vi "Orca Flash Engine.vi"(0 "Notifier Name":string, 11 "Camera ID":string[](array[string])) -> ()   [LabVIEW 2016]
uses:
  Orca Flash Controls/Orca Flash Parameters.ctl
  Orca Flash Controls/Orca Flash Parameter List.ctl
  Orca Flash Controls/Orca Flash ROI.ctl
  Orca Flash Controls/Orca Flash Notifier Element.ctl
  Orca Flash Controls/Orca Flash Actions.ctl
  <vilib>/vision/Image Controls.llb/IMAQ Image.ctl
  Camera Controls/Camera IMAQ Key Info.ctl
panel:
  in  "Orca Flash ROI":T1
  in  "Use Display Module":bool
  in  "Sensor Mode":enum32{"Area", "Progressive"}(radio)
  in  "Number of lines":dbl=8.0
  in  "Internal Line Interval Setpoint":dbl=0.001
  in  "Get Parameter":bool
  in  "Set Parameter":bool
  in  "Get ROI":bool
  in  "Set ROI":bool
  in  "sCMOS Parameter":T2={"Value"=0.0, "Parameter"=2049184} {"Parameter" items=["SENSOR MODE"=4212128, "READOUT SPEED"=4211872, "READOUT DIRECTION"=4211904, "TRIGGER GLOBAL EXPOSURE"=2049680, "TRIGGER DELAY"=1066480, "SYNC READOUT SYSTEM BLANK"=1066528, "SENSOR COOLER"=2115248, "SENSOR COOLER STATUS"=2115280, "EXPOSURE TIME"=2049184, "DEFECT CORRECT MODE"=4670368, "BINNING"=4215968, "INTERNAL LINE SPEED"=4226000, "INTERNAL LINE INTERVAL"=4226016, "IMAGE PIXEL TYPE"=4343296, "NUMBER OF OUTPUT TRIGGER CONNECTOR"=1852320, "OUTPUT TRIGGER SOURCE[0]"=1852576, "OUTPUT TRIGGER SOURCE[1]"=1852832, "OUTPUT TRIGGER SOURCE[2]"=1853088, "OUTPUT TRIGGER POLARITY[0]"=1852592, "OUTPUT TRIGGER POLARITY[1]"=1852848, "OUTPUT TRIGGER POLARITY[2]"=1853104, "OUTPUT TRIGGER ACTIVE[0]"=1852608, "OUTPUT TRIGGER ACTIVE[1]"=1852864, "OUTPUT TRIGGER ACTIVE[2]"=1853120, "OUTPUT TRIGGER DELAY[0]"=1852624, "OUTPUT TRIGGER DELAY[1]"=1852880, "OUTPUT TRIGGER DELAY[2]"=1853136, "OUTPUT TRIGGER PERIOD[0]"=1852640, "OUTPUT TRIGGER PERIOD[1]"=1852896, "OUTPUT TRIGGER PERIOD[2]"=1853152, "OUTPUT TRIGGER KIND[0]"=1852656, "OUTPUT TRIGGER KIND[1]"=1852912, "OUTPUT TRIGGER KIND[2]"=1853168, "OUTPUT TRIGGER PRE HSYNC COUNT"=1852704]}
  in  "# of frames":i32=100
  in  "Path":path
  in  "RECORD":bool
  in  "PREVIEW":bool
  out "Acquisition Loop":i32
  in  "QUIT":bool
  out "Acquisition Frame":i32
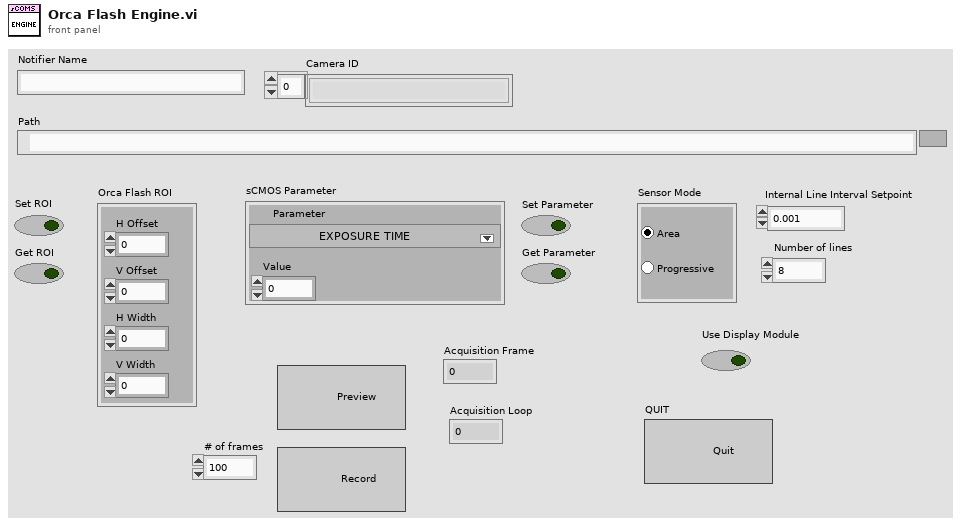
[diagram p1: front panel]
types:
  T1 = typedef "Orca Flash ROI.ctl" = cluster{"H Offset":i32, "V Offset":i32, "H Width":i32, "V Width":i32}
  T2 = typedef "Orca Flash Parameters.ctl" = cluster{"Value":dbl, "Parameter":T3}
  T3 = typedef "Orca Flash Parameter List.ctl" = u32
  T4 = typedef "Camera IMAQ Key Info.ctl" = cluster{"Frame":u32, "Sensor Height":i32, "Sensor Width":i32, "ROI Height":i32, "ROI Width":i32, "ROI Enable?":bool, "Bit per Pixel":u8}
  T5 = typedef "Image Type" = u32
  T6 = typedef "Orca Flash Notifier Element.ctl" = cluster{"Camera Actions":T7, "Received?":bool, "Running?":bool, "sCMOS Parameter":T2, "sCMOS ROI":T1, "Save Path":path, "# of frames":u32, "Image Ref":T8}
  T7 = typedef "Orca Flash Actions.ctl" = enum16{"IDLE", "PREVIEW", "RECORD", "Record Settings", "SETPARAM", "GETPARAM", "SETROI", "GETROI", "PROGRESSIVE MODE", "AREA MODE", "STATUS", "QUIT"}
  T8 = typedef "IMAQ Image.ctl" = refnum<image>
  T9 = enum32{"Invalid", "Standard", "Closed", "Hidden", "Minimized", "Maximized"}
  T10 = cluster{"Horizontal Offset":i32, "Vertical Offset":i32, "Horizontal Size":i32, "Vertical Size":i32}
  T11 = typedef "LVMinMaxIncTypeDef.ctl" = cluster{"Minimum":dbl, "Maximum":dbl, "Increment":dbl}
  T12 = cluster{"H Offset":cluster{"Value":i32, "Limits":T11}, "V Offset":cluster{"Value":i32, "Limits":T11}, "H Size":cluster{"Value":i32, "Limits":T11}, "V Size":cluster{"Value":i32, "Limits":T11}}
  T13 = cluster{"Input Trigger Mode":u32, "Input Trigger Polarity":u32, "Times":u32, "Delay":dbl}
  T14 = cluster{"Output Trigger Period":dbl, "Delay":dbl, "Source":u32}
  T15 = cluster{"Output Trigger Mode":u32, "Output Trigger Polarity":u32}
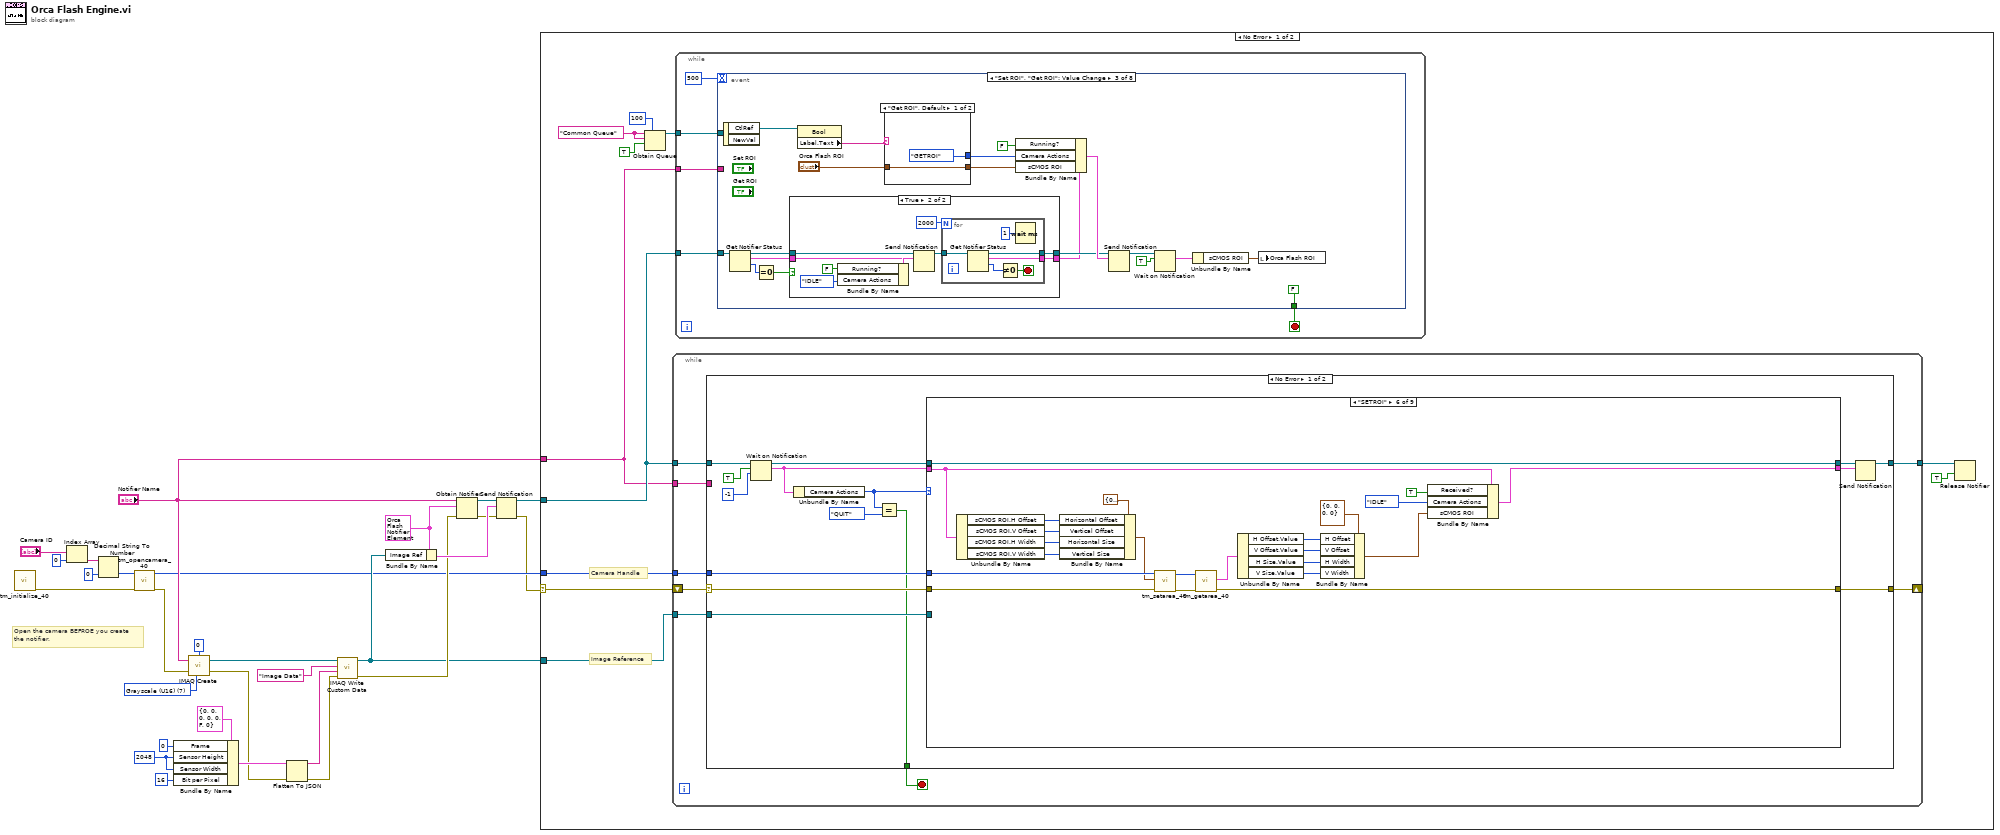
[diagram p0: block diagram]
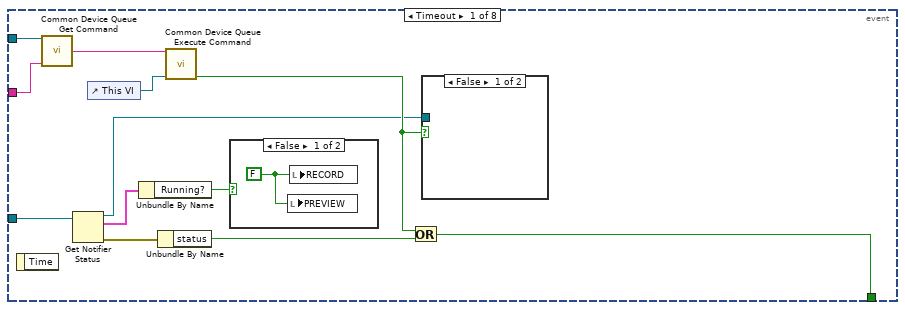
[diagram p2: hidden frame]
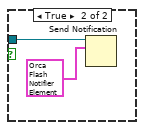
[diagram p3: hidden frame]
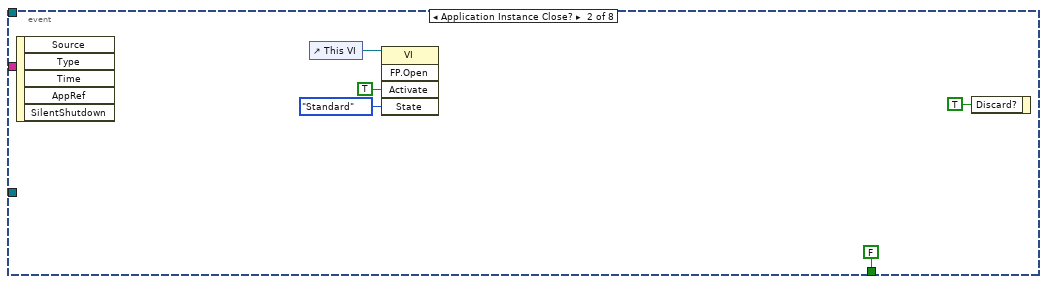
[diagram p5: hidden frame]
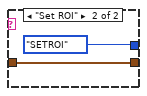
[diagram p7: hidden frame]
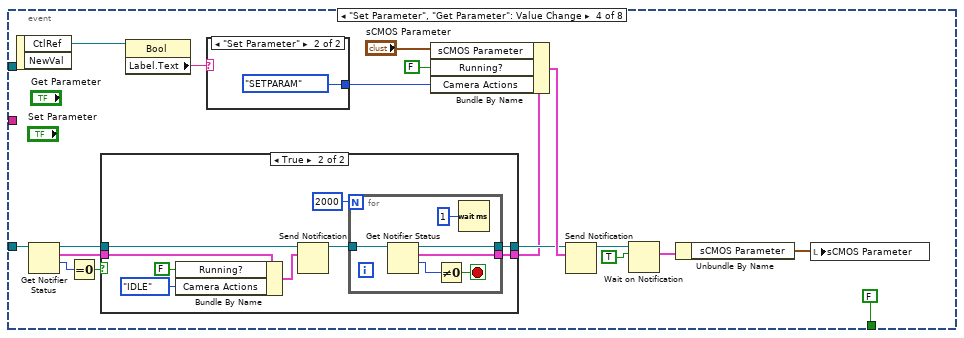
[diagram p8: hidden frame]
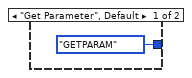
[diagram p10: hidden frame]
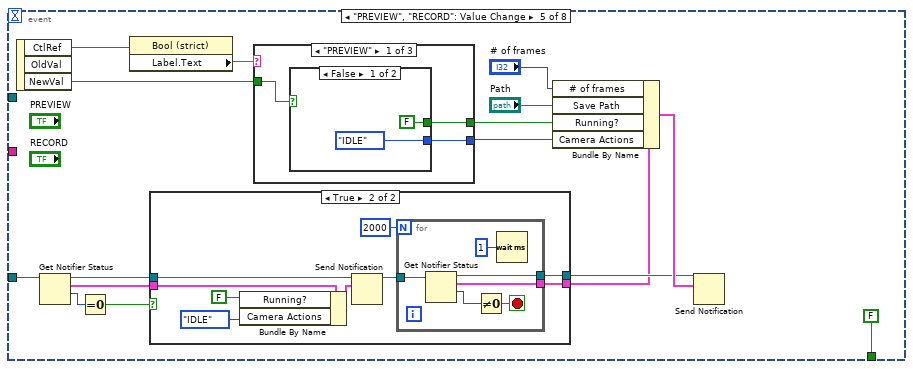
[diagram p11: hidden frame]
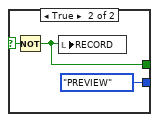
[diagram p13: hidden frame]
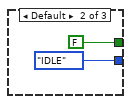
[diagram p14: hidden frame]
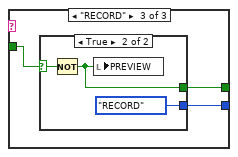
[diagram p15: hidden frame]
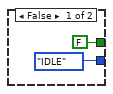
[diagram p16: hidden frame]
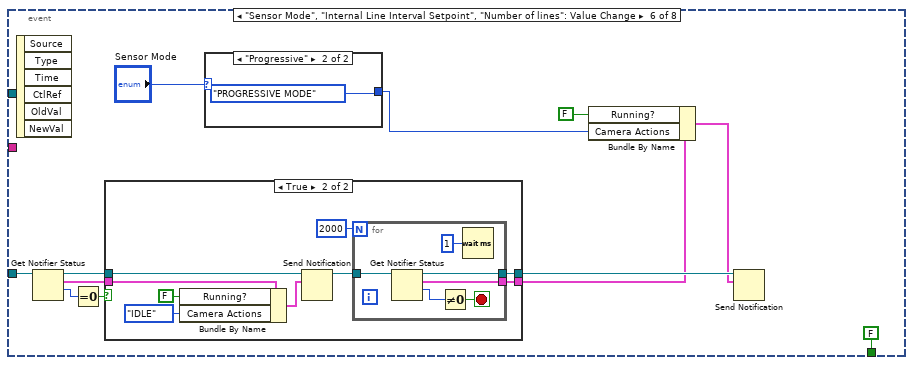
[diagram p17: hidden frame]
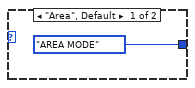
[diagram p18: hidden frame]
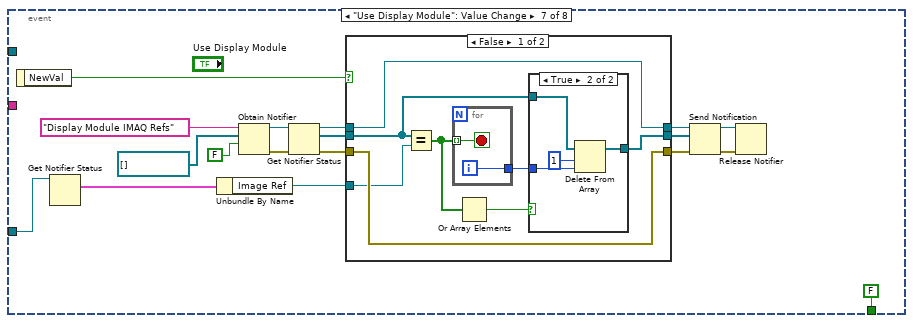
[diagram p20: hidden frame]
diagram:
  w14 = 2048 ("Sensor Height")
  w10 = T5 7 items=["Grayscale (U8)", "Grayscale (I16)", "Grayscale (SGL)", "Complex (CSG)", "RGB (U32)", "HSL (U32)", "RGB (U64)", "Grayscale (U16)"] ("Image Type")
  w24 = T6 {"Camera Actions"=enum."IDLE", "Received?"=FALSE, "Running?"=FALSE, "sCMOS Parameter"={"Value"=0.0, "Parameter"=0}, "sCMOS ROI"={"H Offset"=0, "V Offset"=0, "H Width"=0, "V Width"=0}, "Save Path"=path "", "# of frames"=1, "Image Ref"=refnum} ("Camera Cluster")
  # "Open the camera BEFROE you create\nthe notifier."
  n1 = call <userlib>:"tm_initialize_40.vi"() -> ("error out"=w21:errorcluster)  [unwired: 8 in, 3 out]
  n2 = Index Array(array="Camera ID", index=0) -> (element=w27:string)
  n3 = Decimal String To Number(string=w27, default (0L)=u32 0 ("default (0 I32)")) -> (number=w20:u32)  [unwired: 1 in, 1 out]
  n4 = call <userlib>:"tm_opencamera_40.vi"("error in (no error)"=w21, "Camera Index"=w20) -> ("error out"=w2:errorcluster, "Handle out"=w3:u32)  [unwired: 7 in, 1 out]
  n5 = Bundle By Name(cluster=T4 {"Frame"=0, "Sensor Height"=0, "Sensor Width"=0, "ROI Height"=0, "ROI Width"=0, "ROI Enable?"=FALSE, "Bit per Pixel"=0} ("Camera IMAQ Key Info"), "Frame"=u32 0, "Sensor Height"=w14, "Sensor Width"=w14, "Bit per Pixel"=u8 16) -> (w17:T4)
  n6 = call "IMAQ Create"("Border Size"=0, "Image Name"="Notifier Name", "Image Type"=w10, "error in (no error)"=w2) -> ("New Image"=w12:T8, "error out"=w9:errorcluster)  [unwired: 1 in]
  n7 = Flatten To JSON(anything=w17, error in (no error)=w9) -> (JSON string=w18:string, 11:w8:errorcluster)  [unwired: 1 in]
  n8 = call "IMAQ Write Custom Data"("error in (no error)"=w8, "Custom Data In"=w18, "Key"="Image Data", "Image"=w12) -> ("error out"=w7:errorcluster, "Image Out"=w4:T8)  [unwired: 6 in]
  n9 = Bundle By Name(cluster=w24, "Image Ref"=w4) -> (w25:T6)
  n10 = Obtain Notifier(name (unnamed)="Notifier Name", notification data type=w24, error in (no error)=w7) -> (notifier out=w23:refnum<notifier>, error out=w22:errorcluster)  [unwired: 1 in, 1 out]
  n11 = Send Notification(notification=w25, notifier=w23, error in (no error)=w22) -> (notifier out=w6:refnum<notifier>, error out=w1:errorcluster)
  n12 = case shown="No Error" w1 {
    selector: w1 -> [w35 w591]
    tunnel: w6 -> [w33 w584]
    tunnel: "Notifier Name" -> [w30 w581]
    tunnel: w4 -> [w36 _]
    tunnel: w3 -> [w34 _]
    frame No Error {
      w40 = "Common Queue" ("Unique Notifier Name")
      # "Image Reference"
      # "Camera Handle"
      n13 = Obtain Queue(max queue size (-1, unlimited)=100, name (unnamed)=w40, element data type=w40, create if not found? (T)=TRUE) -> (queue out=w37:refnum<queue>)  [unwired: 1 in, 2 out]
      n14 = while {
        tunnel: w33 -> [w298]
        tunnel: w36 -> [w297]
        shift-right: [w295] -> _
        shift-left: w35 -> [w294]
        tunnel: w34 -> [w296]
        tunnel: [w293] -> w31
        tunnel: w30 -> [w291]
        stop <- w292 stop-if-true
        n15 = case shown="No Error" w294 {
          selector: w294 -> [w303 w572]
          tunnel: w298 -> [w313 w580]
          tunnel: w297 -> [w312 _]
          tunnel: [w302 w580] -> w293
          tunnel: w296 -> [w305 _]
          tunnel: [w304 errorcluster {"status"=FALSE, "code"=0, "source"=""} ("error out")] -> w295
          tunnel: [w299 FALSE] -> w292
          tunnel: w291 -> [_ w571]
          frame No Error {
            n16 = Wait on Notification(notifier=w313, ignore previous (F)=TRUE, timeout in ms (-1)=-1) -> (notifier out=w308:refnum<notifier>, notification=w307:T6)  [unwired: 1 in, 2 out]
            n17 = Unbundle By Name(w307) -> ("Camera Actions"=w301:T7)
            n18 = Equal?(x=w301, y=Orca_Flash_Actions."QUIT") -> (x = y?=w299:bool)
            n19 = case shown="\"SETROI\"" w301 {
              selector: w301 -> [_ w321 _ _ _ _ _ _ _]
              tunnel: w305 -> [_ w346 w423 w439 w452 w475 w486 w507 w561]
              tunnel: w303 -> [w318 w325 w424 w438 w451 w474 w485 w506 w560]
              tunnel: [w318 w330 w422 w434 w450 w467 w484 w494 w550] -> w304
              tunnel: w308 -> [w317 w353 w430 w443 w453 w476 w491 w521 w570]
              tunnel: w312 -> [_ w344 w425 _ _ _ _ _ _]
              tunnel: w307 -> [w315 w342 w428 w437 w448 w470 w488 w518 w557]
              tunnel: [w317 w343 w430 w443 w453 w476 w491 w521 w570] -> w309
              tunnel: [w314 w338 w427 w442 w444 w469 w487 w517 w556] -> w306
              frame "IDLE", Default {
                w316 = FALSE ("Running?")
                n20 = Bundle By Name(cluster=w315, "Received?"=w316, "Running?"=w316) -> (w314:T6)
              }
              frame "PREVIEW", "RECORD" {
                w319 = TRUE ("Running?")
                w350 = 1 items=["Snap", "Sequence"] ("Capture mode")
                n21 = Unbundle By Name(w342) -> ("# of frames"=w331:u32, "Save Path"=w328:path)
                n22 = Equal?(x=w321, y=Orca_Flash_Actions."RECORD") -> (x = y?=w320:bool)
                n23 = To Long Integer(number=w331) -> (32bit integer=w326:i32)
                n24 = call <userlib>:"tm_preparecapture_40.vi"("error in (no error)"=w325, "Capture mode"=w350, "Handle in"=w346) -> ("error out"=w352:errorcluster, "Handle out"=w351:u32)  [unwired: 5 in, 2 out]
                n25 = call "Orca Flash Sort Filenames.vi"("Requested File Path"=w328) -> ("Resulting File Path"=w327:path)  [unwired: 14 in]
                n26 = case shown="True" w320 {
                  tunnel: w352 -> [w355 w361]
                  tunnel: w351 -> [w354 w360]
                  tunnel: [w354 w359] -> w337
                  tunnel: [w355 w358] -> w335
                  tunnel: w327 -> [_ w357]
                  tunnel: w326 -> [_ w356]
                  frame False {
                  }
                  frame True {
                    n27 = call <userlib>:"tm_startrecorder_40.vi"("error in (no error)"=w361, "frames"=w356, "File"=w357, "Handle in"=w360) -> ("error out"=w358:errorcluster, "Handle out"=w359:u32)  [unwired: 6 in]
                  }
                }
                n28 = Bundle By Name(cluster=w342, "Running?"=w319, "Received?"=w319) -> (w341:T6)
                n29 = call <userlib>:"tm_startcapture_40.vi"("error in (no error)"=w335, "Handle in"=w337) -> ("error out"=w324:errorcluster, "Handle out"=w336:u32)  [unwired: 8 in]
                n30 = Send Notification(notification=w341, notifier=w353, error in (no error)=w324) -> (notifier out=w345:refnum<notifier>, error out=w323:errorcluster)
                n31 = case shown="No Error" w323 {
                  selector: w323 -> [w369 w419]
                  tunnel: [w377 w420] -> w349
                  tunnel: w345 -> [w376 w421]
                  tunnel: w344 -> [w375 _]
                  tunnel: [w374 w418] -> w343
                  tunnel: [w373 w417] -> w340
                  tunnel: w336 -> [w372 w420]
                  tunnel: [w371 w419] -> w334
                  tunnel: w326 -> [w370 _]
                  tunnel: w320 -> [w368 _]
                  frame No Error {
                    n32 = while {
                      tunnel: w370 -> [w405]
                      tunnel: w376 -> [w408]
                      tunnel: [w407] -> w374
                      tunnel: w375 -> [w404]
                      tunnel: [w402] -> w373
                      tunnel: w369 -> [w411]
                      tunnel: [w379] -> w371
                      tunnel: w372 -> [w412]
                      tunnel: [w400] -> w377
                      tunnel: w368 -> [w378]
                      i -> [w406]
                      stop <- w409 stop-if-true
                      w385 = "Image Data" ("Key")
                      n33 = call <userlib>:"tm_waitnextframe_40.vi"("error in (no error)"=w411, "Handle in"=w412) -> ("error out"=w396:errorcluster, "Frame Count"=w394:i32, "Frame Index"=w399:i32, "Handle out"=w410:u32)  [unwired: 6 in]
                      "Acquisition Frame" <- w394
                      n34 = call <userlib>:"tm_getframe16_40.vi"("error in (no error)"=w396, "Frame Index"=w399, "Handle in"=w410) -> ("error out"=w384:errorcluster, "Data"=w395:u16[][], "Handle out"=w400:u32)  [unwired: 5 in, 1 out]
                      n35 = case shown="False" w378 {
                        selector: w378 -> [w413 _]
                        tunnel: w405 -> [_ w416]
                        tunnel: [w413 w415] -> w397
                        tunnel: w394 -> [_ w414]
                        frame False {
                        }
                        frame True {
                          n36 = Greater Or Equal?(x=w414, y=w416) -> (x >= y?=w415:bool)
                        }
                      }
                      n37 = To Unsigned Long Integer(number=w394) -> (unsigned 32bit integer=w388:u32)
                      n38 = call "IMAQ ArrayToImage"("Image Pixels (U16)"=w395, "error in (no error)"=w384, "Image"=w404) -> ("error out"=w383:errorcluster, "Image Out"=w393:T8)  [unwired: 7 in]
                      n39 = call "IMAQ Read Custom Data"("error in (no error)"=w383, "Key"=w385, "Image"=w393) -> ("error out"=w382:errorcluster, "Custom Data Out"=w390:string, "Image (duplicate)"=w392:T8)  [unwired: 6 in]
                      n40 = Unflatten From JSON(JSON string=w390, type and defaults=T4 {"Frame"=0, "Sensor Height"=0, "Sensor Width"=0, "ROI Height"=0, "ROI Width"=0, "ROI Enable?"=FALSE, "Bit per Pixel"=0} ("Camera IMAQ Key Info"), error in (no error)=w382) -> (value=w389:T4, error out=w381:errorcluster)  [unwired: 4 in]
                      n41 = Bundle By Name(cluster=w389, "Frame"=w388) -> (w387:T4)
                      n42 = Get Notifier Status(notifier=w408) -> (notifier out=w407:refnum<notifier>, current notification=w402:T6)  [unwired: 1 in, 3 out]
                      n43 = Flatten To JSON(anything=w387, error in (no error)=w381) -> (JSON string=w386:string, 11:w380:errorcluster)  [unwired: 1 in]
                      n44 = Unbundle By Name(w402) -> ("Running?"=w403:bool)
                      n45 = call "IMAQ Write Custom Data"("error in (no error)"=w380, "Custom Data In"=w386, "Key"=w385, "Image"=w392) -> ("error out"=w379:errorcluster)  [unwired: 6 in, 1 out]
                      n46 = Unbundle By Name(w379) -> ("status"=w398:bool)
                      n47 = Not(x=w403) -> (.not. x?=w401:bool)
                      n48 = Compound Arithmetic op=OR(w401, w397, w398) -> (w409:bool)
                      "Acquisition Loop" <- w406
                    }
                  }
                  frame Error {
                    n49 = Get Notifier Status(notifier=w421) -> (notifier out=w418:refnum<notifier>, current notification=w417:T6)  [unwired: 1 in, 3 out]
                  }
                }
                n50 = call <userlib>:"tm_stopcapture_40.vi"("error in (no error)"=w334, "Handle in"=w349) -> ("error out"=w333:errorcluster, "Handle out"=w348:u32)  [unwired: 8 in]
                n51 = case shown="False" w320 {
                  tunnel: w348 -> [w363 w367]
                  tunnel: [w363 w366] -> w347
                  tunnel: w333 -> [w362 w365]
                  tunnel: [w362 w364] -> w332
                  frame False {
                  }
                  frame True {
                    n52 = call <userlib>:"tm_stoprecorder_40.vi"("error in (no error)"=w365, "Handle in"=w367) -> ("error out"=w364:errorcluster, "Handle out"=w366:u32)  [unwired: 8 in]
                  }
                }
                n53 = Bundle By Name(cluster=w340, "Running?"=FALSE, "Camera Actions"=Orca_Flash_Actions."IDLE") -> (w338:T6)
                n54 = call <userlib>:"tm_unpreparecapture_40.vi"("error in (no error)"=w332, "Handle in"=w347) -> ("error out"=w330:errorcluster)  [unwired: 8 in, 1 out]
              }
              frame "QUIT" {
                n55 = call <userlib>:"tm_closecamera_40.vi"("error in (no error)"=w424, "Handle in"=w423) -> ("error out"=w426:errorcluster)  [unwired: 9 in]
                n56 = call "IMAQ Dispose"("Image"=w425) -> ()  [unwired: 5 in, 1 out]
                n57 = Bundle By Name(cluster=w428, "Received?"=TRUE ("Running?")) -> (w427:T6)
                n58 = call <userlib>:"tm_deinitialize_40.vi"("error in (no error)"=w426) -> ("error out"=w422:errorcluster)  [unwired: 10 in]
              }
              frame "SETPARAM" {
                n59 = Unbundle By Name(w437) -> ("sCMOS Parameter.Parameter"=w432:T3, "sCMOS Parameter.Value"=w436:dbl)
                n60 = call <userlib>:"tm_setparameter_40.vi"("error in (no error)"=w438, "Value in"=w436, "Parameter"=w432, "Handle in"=w439) -> ("error out"=w435:errorcluster, "Handle out"=w433:u32)  [unwired: 6 in]
                n61 = call <userlib>:"tm_getparameter_40.vi"("error in (no error)"=w435, "Parameter"=w432, "Handle in"=w433) -> ("error out"=w434:errorcluster, "Value out"=w431:dbl)  [unwired: 6 in, 1 out]
                n62 = Bundle By Name(cluster=w437, "Received?"=TRUE ("Running?"), "Camera Actions"=Orca_Flash_Actions."IDLE", "sCMOS Parameter.Value"=w431) -> (w442:T6)
              }
              frame "GETPARAM" {
                n63 = Unbundle By Name(w448) -> ("sCMOS Parameter.Parameter"=w449:T3)
                n64 = call <userlib>:"tm_getparameter_40.vi"("error in (no error)"=w451, "Parameter"=w449, "Handle in"=w452) -> ("error out"=w450:errorcluster, "Value out"=w445:dbl)  [unwired: 6 in, 1 out]
                n65 = Bundle By Name(cluster=w448, "Received?"=TRUE ("Running?"), "Camera Actions"=Orca_Flash_Actions."IDLE", "sCMOS Parameter.Value"=w445) -> (w444:T6)
              }
              frame "SETROI" {
                n66 = Unbundle By Name(w470) -> ("sCMOS ROI.H Offset"=w455:i32, "sCMOS ROI.V Offset"=w456:i32, "sCMOS ROI.H Width"=w457:i32, "sCMOS ROI.V Width"=w458:i32)
                n67 = Bundle By Name(cluster=T10 {"Horizontal Offset"=0, "Vertical Offset"=0, "Horizontal Size"=0, "Vertical Size"=0} ("Sub Region"), "Horizontal Offset"=w455, "Vertical Offset"=w456, "Horizontal Size"=w457, "Vertical Size"=w458) -> (w454:T10)
                n68 = call <userlib>:"tm_setarea_40.vi"("error in (no error)"=w474, "Sub Region"=w454, "Handle in"=w475) -> ("error out"=w468:errorcluster, "Handle out"=w473:u32)  [unwired: 7 in]
                n69 = call <userlib>:"tm_getarea_40.vi"("error in (no error)"=w468, "Handle in"=w473) -> ("error out"=w467:errorcluster, "Sub Region"=w466:T12)  [unwired: 7 in, 1 out]
                n70 = Unbundle By Name(w466) -> ("H Offset.Value"=w464:i32, "V Offset.Value"=w463:i32, "H Size.Value"=w462:i32, "V Size.Value"=w461:i32)
                n71 = Bundle By Name(cluster=T1 {"H Offset"=0, "V Offset"=0, "H Width"=0, "V Width"=0} ("Orca Flash ROI"), "H Offset"=w464, "V Offset"=w463, "H Width"=w462, "V Width"=w461) -> (w460:T1)
                n72 = Bundle By Name(cluster=w470, "Received?"=TRUE ("Running?"), "Camera Actions"=Orca_Flash_Actions."IDLE", "sCMOS ROI"=w460) -> (w469:T6)
              }
              frame "GETROI" {
                n73 = call <userlib>:"tm_getarea_40.vi"("error in (no error)"=w485, "Handle in"=w486) -> ("error out"=w484:errorcluster, "Sub Region"=w483:T12)  [unwired: 7 in, 1 out]
                n74 = Unbundle By Name(w483) -> ("H Offset.Value"=w478:i32, "V Offset.Value"=w479:i32, "H Size.Value"=w480:i32, "V Size.Value"=w481:i32)
                n75 = Bundle By Name(cluster=T1 {"H Offset"=0, "V Offset"=0, "H Width"=0, "V Width"=0} ("Orca Flash ROI"), "H Offset"=w478, "V Offset"=w479, "H Width"=w480, "V Width"=w481) -> (w477:T1)
                n76 = Bundle By Name(cluster=w488, "Received?"=TRUE ("Running?"), "Camera Actions"=Orca_Flash_Actions."IDLE", "sCMOS ROI"=w477) -> (w487:T6)
              }
              frame "PROGRESSIVE MODE" {
                w493 = u32 2049184 items=["SENSOR MODE"=4212128, "READOUT SPEED"=4211872, "READOUT DIRECTION"=4211904, "TRIGGER GLOBAL EXPOSURE"=2049680, "TRIGGER DELAY"=1066480, "INTERNAL TRIGGER HANDLING"=1066496, "SYNC READOUT SYSTEM BLANK"=1066528, "SENSOR TEMPERATURE"=2115232, "SENSOR COOLER STATUS"=2115280, "EXPOSURE TIME"=2049184, "DEFECT CORRECT MODE"=4670368, "BINNING"=4215968, "INTERNAL LINE SPEED"=4226000, "INTERNAL LINE INTERVAL"=4226016, "NUMBER OF OUTPUT TRIGGER CONNECTOR"=1852320, "OUTPUT TRIGGER SOURCE[0]"=1852576, "OUTPUT TRIGGER SOURCE[1]"=1852832, "OUTPUT TRIGGER SOURCE[2]"=1853088, "OUTPUT TRIGGER POLARITY[0]"=1852592, "OUTPUT TRIGGER POLARITY[1]"=1852848, "OUTPUT TRIGGER POLARITY[2]"=1853104, "OUTPUT TRIGGER ACTIVE[0]"=1852608, "OUTPUT TRIGGER ACTIVE[1]"=1852864, "OUTPUT TRIGGER ACTIVE[2]"=1853120, "OUTPUT TRIGGER DELAY[0]"=1852624, "OUTPUT TRIGGER DELAY[1]"=1852880, "OUTPUT TRIGGER DELAY[2]"=1853136, "OUTPUT TRIGGER PERIOD[0]"=1852640, "OUTPUT TRIGGER PERIOD[1]"=1852896, "OUTPUT TRIGGER PERIOD[2]"=1853152, "OUTPUT TRIGGER KIND[0]"=1852656, "OUTPUT TRIGGER KIND[1]"=1852912, "OUTPUT TRIGGER KIND[2]"=1853168, "OUTPUT TRIGGER BASE SENSOR[0]"=1852672, "OUTPUT TRIGGER BASE SENSOR[1]"=1852928, "OUTPUT TRIGGER BASE SENSOR[2]"=1853184, "OUTPUT TRIGGER PRE HSYNC COUNT"=1852704] ("Parameter")
                w499 = u32 4226016 items=["SENSOR MODE"=4212128, "READOUT SPEED"=4211872, "READOUT DIRECTION"=4211904, "TRIGGER GLOBAL EXPOSURE"=2049680, "TRIGGER DELAY"=1066480, "INTERNAL TRIGGER HANDLING"=1066496, "SYNC READOUT SYSTEM BLANK"=1066528, "SENSOR TEMPERATURE"=2115232, "SENSOR COOLER STATUS"=2115280, "EXPOSURE TIME"=2049184, "DEFECT CORRECT MODE"=4670368, "BINNING"=4215968, "INTERNAL LINE SPEED"=4226000, "INTERNAL LINE INTERVAL"=4226016, "NUMBER OF OUTPUT TRIGGER CONNECTOR"=1852320, "OUTPUT TRIGGER SOURCE[0]"=1852576, "OUTPUT TRIGGER SOURCE[1]"=1852832, "OUTPUT TRIGGER SOURCE[2]"=1853088, "OUTPUT TRIGGER POLARITY[0]"=1852592, "OUTPUT TRIGGER POLARITY[1]"=1852848, "OUTPUT TRIGGER POLARITY[2]"=1853104, "OUTPUT TRIGGER ACTIVE[0]"=1852608, "OUTPUT TRIGGER ACTIVE[1]"=1852864, "OUTPUT TRIGGER ACTIVE[2]"=1853120, "OUTPUT TRIGGER DELAY[0]"=1852624, "OUTPUT TRIGGER DELAY[1]"=1852880, "OUTPUT TRIGGER DELAY[2]"=1853136, "OUTPUT TRIGGER PERIOD[0]"=1852640, "OUTPUT TRIGGER PERIOD[1]"=1852896, "OUTPUT TRIGGER PERIOD[2]"=1853152, "OUTPUT TRIGGER KIND[0]"=1852656, "OUTPUT TRIGGER KIND[1]"=1852912, "OUTPUT TRIGGER KIND[2]"=1853168, "OUTPUT TRIGGER BASE SENSOR[0]"=1852672, "OUTPUT TRIGGER BASE SENSOR[1]"=1852928, "OUTPUT TRIGGER BASE SENSOR[2]"=1853184, "OUTPUT TRIGGER PRE HSYNC COUNT"=1852704] ("Parameter")
                w510 = u32 1 items=["FORWARD"=1, "BACKWARD"=2] ("Readout Direction")
                w514 = u32 4212128 items=["SENSOR MODE"=4212128, "CCD MODE"=4212384, "READOUT MODE"=4211872, "ACTIVE VIEW INDEX"=4343136, "BITS PER CHANNEL"=4342976, "IMAGE PIXEL TYPE"=4343296, "BINNING"=4215968, "EXPOSURE TIME"=2049184, "CONTRAST GAIN"=3163312, "CONTRAST OFFSET"=3163328, "LIGHT MODE"=2114720, "SENSITIVITY"=2114992, "PHOTON IMAGING MODE"=2115200, "HIGH DYNAMIC RANGE MODE"=3163360, "WHITE BALANCE"=3163568, "TEMPERATURE"=2115232, "TEMPERATURE TARGET"=2115264, "SENSOR COOLER FAN"=2115296, "LINEBUNDLE HEIGHT"=4212192, "MECHANICAL SHUTTER"=2115488, "BACK FOCUS POSITION"=8422304, "TRIGGER CONNECTOR"=1066432, "TRIGGER SOURCE"=1066144, "OUTPUT TRIGGER SOURCE"=1852576, "TRIGGER GLOBAL EXPOSURE"=2049680, "FIRST TRIGGER BEHAVIOR"=2049696, "CHANNEL SYNC"=1852352, "READOUT DIRECTION"=4211904, "PRE HSYNC COUNT"=1852704, "INTERNAL LINE SPEED"=4191408, "INTERNAL LINE INTERVAL"=4191424] ("Parameter")
                w513 = u32 4211904 items=["SENSOR MODE"=4212128, "CCD MODE"=4212384, "READOUT MODE"=4211872, "ACTIVE VIEW INDEX"=4343136, "BITS PER CHANNEL"=4342976, "IMAGE PIXEL TYPE"=4343296, "BINNING"=4215968, "EXPOSURE TIME"=2049184, "CONTRAST GAIN"=3163312, "CONTRAST OFFSET"=3163328, "LIGHT MODE"=2114720, "SENSITIVITY"=2114992, "PHOTON IMAGING MODE"=2115200, "HIGH DYNAMIC RANGE MODE"=3163360, "WHITE BALANCE"=3163568, "TEMPERATURE"=2115232, "TEMPERATURE TARGET"=2115264, "SENSOR COOLER FAN"=2115296, "LINEBUNDLE HEIGHT"=4212192, "MECHANICAL SHUTTER"=2115488, "BACK FOCUS POSITION"=8422304, "TRIGGER CONNECTOR"=1066432, "TRIGGER SOURCE"=1066144, "OUTPUT TRIGGER SOURCE"=1852576, "TRIGGER GLOBAL EXPOSURE"=2049680, "FIRST TRIGGER BEHAVIOR"=2049696, "CHANNEL SYNC"=1852352, "READOUT DIRECTION"=4211904, "PRE HSYNC COUNT"=1852704, "INTERNAL LINE SPEED"=4191408, "INTERNAL LINE INTERVAL"=4191424] ("Parameter")
                n77 = case shown="\"Master\"" enum16{"Master", "Slave"}."Master" ("Camera Trigger Mode") {
                  tunnel: [w525 w541] -> w512
                  tunnel: [w524 w539] -> w511
                  tunnel: w507 -> [w523 w543]
                  tunnel: w506 -> [w522 w542]
                  frame "Slave", Default {
                    w530 = u32 2 items=["NEGATIVE"=1, "POSITIVE"=2] ("Input Trigger Polarity")
                    w529 = u32 2 items=["INTERNAL"=1, "EXTERNAL EDGE"=2, "EXTERNAL LEVEL"=4, "SOFTWARE"=32, "FAST REPETITION"=64, "TDI"=128, "START"=512, "SYNC READOUT"=1024] ("Input Trigger Mode")
                    n78 = Bundle("Input Trigger Mode"=w529, "Input Trigger Polarity"=w530, "Times"=u32 1, "Delay"=0.0) -> (w526:T13)  [unwired: 1 in]
                    n79 = call <userlib>:"tm_setinputtrigger_40.vi"("error in (no error)"=w522, "Parameters"=w526, "Handle in"=w523) -> ("error out"=w524:errorcluster, "Handle out"=w525:u32)  [unwired: 7 in]
                  }
                  frame "Master" {
                    w536 = u32 2 items=["Exposure"=1, "Readout End"=2, "V Sync"=3, "H Sync"=4, "Trigger"=6] ("Source")
                    w538 = u32 2 items=["NEGATIVE"=1, "POSITIVE"=2] ("Output Trigger Polarity")
                    w537 = u32 3 items=["LOW"=1, "GLOBAL EXPOSURE"=2, "PROGRAMMABLE"=3, "TRIGGER READY"=4, "HIGH"=5] ("Output Trigger Mode")
                    w549 = u32 2 items=["NEGATIVE"=1, "POSITIVE"=2] ("Input Trigger Polarity")
                    w548 = u32 1 items=["INTERNAL"=1, "EXTERNAL EDGE"=2, "EXTERNAL LEVEL"=4, "SOFTWARE"=32, "FAST REPETITION"=64, "TDI"=128, "START"=512, "SYNC READOUT"=1024] ("Input Trigger Mode")
                    n80 = Bundle("Input Trigger Mode"=w548, "Input Trigger Polarity"=w549, "Times"=u32 1, "Delay"=0.0) -> (w545:T13)  [unwired: 1 in]
                    n81 = call <userlib>:"tm_setinputtrigger_40.vi"("error in (no error)"=w542, "Parameters"=w545, "Handle in"=w543) -> ("error out"=w540:errorcluster, "Handle out"=w544:u32)  [unwired: 7 in]
                    n82 = Bundle("Output Trigger Period"=0.001, "Delay"=0.0, "Source"=w536) -> (w533:T14)  [unwired: 1 in]
                    n83 = Bundle("Output Trigger Mode"=w537, "Output Trigger Polarity"=w538) -> (w532:T15)  [unwired: 1 in]
                    n84 = call <userlib>:"tm_setoutputtrigger_40.vi"("Port"=1, "error in (no error)"=w540, "Programmable Options"=w533, "Type"=w532, "Handle in"=w544) -> ("error out"=w539:errorcluster, "Handle out"=w541:u32)  [unwired: 5 in]
                  }
                }
                n85 = Bundle By Name(cluster=w518, "Received?"=TRUE ("Running?"), "Camera Actions"=Orca_Flash_Actions."IDLE") -> (w517:T6)
                n86 = call <userlib>:"tm_setparameter_40.vi"("error in (no error)"=w511, "Value in"=12.0, "Parameter"=w514, "Handle in"=w512) -> ("error out"=w516:errorcluster, "Handle out"=w515:u32)  [unwired: 6 in]
                n87 = To Double Precision Float(number=w510) -> (double precision float=w509:dbl)
                n88 = call <userlib>:"tm_setparameter_40.vi"("error in (no error)"=w516, "Value in"=w509, "Parameter"=w513, "Handle in"=w515) -> ("error out"=w504:errorcluster, "Handle out"=w505:u32)  [unwired: 6 in]
                n89 = call <userlib>:"tm_setparameter_40.vi"("error in (no error)"=w504, "Value in"="Internal Line Interval Setpoint", "Parameter"=w499, "Handle in"=w505) -> ("error out"=w502:errorcluster, "Handle out"=w503:u32)  [unwired: 6 in]
                n90 = call <userlib>:"tm_getparameter_40.vi"("error in (no error)"=w502, "Parameter"=w499, "Handle in"=w503) -> ("error out"=w500:errorcluster, "Value out"=w497:dbl, "Handle out"=w501:u32)  [unwired: 6 in]
                n91 = Multiply(x=w497, y="Number of lines") -> (x*y=w496:dbl)
                n92 = call <userlib>:"tm_setparameter_40.vi"("error in (no error)"=w500, "Value in"=w496, "Parameter"=w493, "Handle in"=w501) -> ("error out"=w494:errorcluster)  [unwired: 6 in, 1 out]
              }
              frame "AREA MODE" {
                w554 = u32 2049184 items=["SENSOR MODE"=4212128, "READOUT SPEED"=4211872, "READOUT DIRECTION"=4211904, "TRIGGER GLOBAL EXPOSURE"=2049680, "TRIGGER DELAY"=1066480, "INTERNAL TRIGGER HANDLING"=1066496, "SYNC READOUT SYSTEM BLANK"=1066528, "SENSOR TEMPERATURE"=2115232, "SENSOR COOLER STATUS"=2115280, "EXPOSURE TIME"=2049184, "DEFECT CORRECT MODE"=4670368, "BINNING"=4215968, "INTERNAL LINE SPEED"=4226000, "INTERNAL LINE INTERVAL"=4226016, "NUMBER OF OUTPUT TRIGGER CONNECTOR"=1852320, "OUTPUT TRIGGER SOURCE[0]"=1852576, "OUTPUT TRIGGER SOURCE[1]"=1852832, "OUTPUT TRIGGER SOURCE[2]"=1853088, "OUTPUT TRIGGER POLARITY[0]"=1852592, "OUTPUT TRIGGER POLARITY[1]"=1852848, "OUTPUT TRIGGER POLARITY[2]"=1853104, "OUTPUT TRIGGER ACTIVE[0]"=1852608, "OUTPUT TRIGGER ACTIVE[1]"=1852864, "OUTPUT TRIGGER ACTIVE[2]"=1853120, "OUTPUT TRIGGER DELAY[0]"=1852624, "OUTPUT TRIGGER DELAY[1]"=1852880, "OUTPUT TRIGGER DELAY[2]"=1853136, "OUTPUT TRIGGER PERIOD[0]"=1852640, "OUTPUT TRIGGER PERIOD[1]"=1852896, "OUTPUT TRIGGER PERIOD[2]"=1853152, "OUTPUT TRIGGER KIND[0]"=1852656, "OUTPUT TRIGGER KIND[1]"=1852912, "OUTPUT TRIGGER KIND[2]"=1853168, "OUTPUT TRIGGER BASE SENSOR[0]"=1852672, "OUTPUT TRIGGER BASE SENSOR[1]"=1852928, "OUTPUT TRIGGER BASE SENSOR[2]"=1853184, "OUTPUT TRIGGER PRE HSYNC COUNT"=1852704] ("Parameter")
                w555 = u32 2 items=["NEGATIVE"=1, "POSITIVE"=2] ("Input Trigger Polarity")
                w569 = u32 1 items=["INTERNAL"=1, "EXTERNAL EDGE"=2, "EXTERNAL LEVEL"=4, "SOFTWARE"=32, "FAST REPETITION"=64, "TDI"=128, "START"=512, "SYNC READOUT"=1024] ("Input Trigger Mode")
                w565 = u32 4212128 items=["SENSOR MODE"=4212128, "CCD MODE"=4212384, "READOUT MODE"=4211872, "ACTIVE VIEW INDEX"=4343136, "BITS PER CHANNEL"=4342976, "IMAGE PIXEL TYPE"=4343296, "BINNING"=4215968, "EXPOSURE TIME"=2049184, "CONTRAST GAIN"=3163312, "CONTRAST OFFSET"=3163328, "LIGHT MODE"=2114720, "SENSITIVITY"=2114992, "PHOTON IMAGING MODE"=2115200, "HIGH DYNAMIC RANGE MODE"=3163360, "WHITE BALANCE"=3163568, "TEMPERATURE"=2115232, "TEMPERATURE TARGET"=2115264, "SENSOR COOLER FAN"=2115296, "LINEBUNDLE HEIGHT"=4212192, "MECHANICAL SHUTTER"=2115488, "BACK FOCUS POSITION"=8422304, "TRIGGER CONNECTOR"=1066432, "TRIGGER SOURCE"=1066144, "OUTPUT TRIGGER SOURCE"=1852576, "TRIGGER GLOBAL EXPOSURE"=2049680, "FIRST TRIGGER BEHAVIOR"=2049696, "CHANNEL SYNC"=1852352, "READOUT DIRECTION"=4211904, "PRE HSYNC COUNT"=1852704, "INTERNAL LINE SPEED"=4191408, "INTERNAL LINE INTERVAL"=4191424] ("Parameter")
                n93 = Bundle("Input Trigger Mode"=w569, "Input Trigger Polarity"=w555, "Times"=u32 1, "Delay"=0.0) -> (w566:T13)  [unwired: 1 in]
                n94 = call <userlib>:"tm_setinputtrigger_40.vi"("error in (no error)"=w560, "Parameters"=w566, "Handle in"=w561) -> ("error out"=w563:errorcluster, "Handle out"=w564:u32)  [unwired: 7 in]
                n95 = Bundle By Name(cluster=w557, "Received?"=TRUE ("Running?"), "Camera Actions"=Orca_Flash_Actions."IDLE") -> (w556:T6)
                n96 = call <userlib>:"tm_setparameter_40.vi"("error in (no error)"=w563, "Value in"=1.0, "Parameter"=w565, "Handle in"=w564) -> ("error out"=w551:errorcluster, "Handle out"=w552:u32)  [unwired: 6 in]
                n97 = call <userlib>:"tm_setparameter_40.vi"("error in (no error)"=w551, "Value in"=0.1, "Parameter"=w554, "Handle in"=w552) -> ("error out"=w550:errorcluster)  [unwired: 6 in, 1 out]
              }
            }
            n98 = Send Notification(notification=w306, notifier=w309) -> (notifier out=w302:refnum<notifier>)  [unwired: 1 in, 1 out]
          }
          frame Error {
            n99 = Unbundle By Name(w572) -> ("source"=w573:string)
            n100 = call <vilib>:"Space Constant.vi"() -> ("String"=w576:string)
            n101 = Concatenate Strings(w571, w576, "Device Error." ("string"), "\r", w573) -> (w577:string)
            n102 = One Button Dialog(message=w577) -> ()  [unwired: 1 in, 1 out]
          }
        }
      }
      n103 = while {
        tunnel: w33 -> [w43]
        tunnel: w37 -> [w42]
        tunnel: w30 -> [w41]
        stop <- w45 stop-if-true
        n104 = event shown="[2] \"Set ROI\", \"Get ROI\": Value Change" {
          selector: _ -> [_ _ _ _ _ _ _ _]
          dyn-events: _ -> [_ _ _ _ _ _ _ _]
          timeout: 500 -> [_ _ _ _ _ _ _ _]
          tunnel: w43 -> [w56 _ w72 w110 w153 w201 w225 w269]
          tunnel: [w52 FALSE ("NewVal") FALSE ("NewVal") FALSE ("NewVal") FALSE ("NewVal") FALSE ("NewVal") FALSE ("NewVal") w273] -> w45
          tunnel: w42 -> [w49 _ _ _ _ _ _ _]
          tunnel: w41 -> [w48 _ _ _ _ _ _ _]
          event Timeout {
            n105 = event-data() -> ()  [unwired: 1 in, 1 out]
            n106 = call "Common Device Queue Get Command.vi"("Common Queue"=w49, "Notifier Name"=w48) -> ("Command"=w51:string)  [unwired: 12 in, 1 out]
            n107 = Get Notifier Status(notifier=w56) -> (notifier out=w46:refnum<notifier>, current notification=w55:T6, error out=w54:errorcluster)  [unwired: 1 in, 2 out]
            n108 = control-ref of="This VI"() -> (w50:refnum<vi>)
            n109 = Unbundle By Name(w55) -> ("Running?"=w57:bool)
            n110 = Unbundle By Name(w54) -> ("status"=w53:bool)
            n111 = call "Common Device Queue Execute Command.vi"("Common Command"=w51, "VI Refnum"=w50) -> ("Quit?"=w47:bool)  [unwired: 12 in, 1 out]
            n112 = case shown="False" w57 {
              frame False {
                w60 = FALSE ("RECORD")
                n113 = local write "PREVIEW"(w60) -> ()
                n114 = local write "RECORD"(w60) -> ()
              }
              frame True {
              }
            }
            n115 = Or(x=w47, y=w53) -> (x .or. y?=w52:bool)
            n116 = case shown="False" w47 {
              tunnel: w46 -> [_ w59]
              frame False {
              }
              frame True {
                n117 = Send Notification(notification=T6 {"Camera Actions"=enum."QUIT", "Received?"=FALSE, "Running?"=FALSE, "sCMOS Parameter"={"Value"=0.0, "Parameter"=0}, "sCMOS ROI"={"H Offset"=0, "V Offset"=0, "H Width"=0, "V Width"=0}, "Save Path"=path "", "# of frames"=1, "Image Ref"=refnum} ("Camera Cluster"), notifier=w59) -> ()  [unwired: 1 in, 2 out]
              }
            }
          }
          event Application Instance Close? {
            n118 = event-data() -> ()  [unwired: 1 in, 5 out]
            n119 = control-ref of="This VI"() -> (w63:refnum<vi>)
            n120 = invoke class="VI" method="FP.Open"(reference=w63, "Activate"=TRUE ("Activate?"), "State"=T9."Standard") -> ()  [unwired: 2 in, 5 out]
            n121 = event-data("Discard?"=TRUE) -> ()  [unwired: 1 in, 1 out]
          }
          event "Set ROI", "Get ROI": Value Change {
            n122 = event-data() -> ("CtlRef"=w82:refnum<vi>)  [unwired: 1 in, 1 out]
            n123 = Get Notifier Status(notifier=w72) -> (notifier out=w70:refnum<notifier>, current notification=w69:T6, # waiting=w68:i32)  [unwired: 1 in, 2 out]
            n124 = Equal To 0?(x=w68) -> (x = 0?=w71:bool)
            n125 = case shown="True" w71 {
              tunnel: [w86 w92] -> w74
              tunnel: [w85 w91] -> w73
              tunnel: w70 -> [w86 w90]
              tunnel: w69 -> [w85 w87]
              frame False {
              }
              frame True {
                n126 = Bundle By Name(cluster=w87, "Running?"=FALSE, "Camera Actions"=Orca_Flash_Actions."IDLE") -> (w94:T6)
                n127 = Send Notification(notification=w94, notifier=w90) -> (notifier out=w95:refnum<notifier>)  [unwired: 1 in, 1 out]
                n128 = for {
                  N: 2000 -> [_]
                  tunnel: w95 -> [w101]
                  tunnel: [w98] -> w92
                  tunnel: [w97] -> w91
                  stop <- w99 stop-if-true
                  n129 = Get Notifier Status(notifier=w101) -> (notifier out=w98:refnum<notifier>, current notification=w97:T6, # waiting=w100:i32)  [unwired: 1 in, 2 out]
                  n130 = Not Equal To 0?(x=w100) -> (x != 0?=w99:bool)
                  n131 = Wait (ms)(milliseconds to wait=u32 1) -> ()  [unwired: 1 out]
                }
              }
            }
            n132 = property class="Bool"(reference=w82) -> ("Label.Text"=w81:string)  [unwired: 1 in, 2 out]
            n133 = case shown="\"Get ROI\", Default" w81 {
              tunnel: [Orca_Flash_Actions."GETROI" ("Camera Actions") Orca_Flash_Actions."SETROI" ("Camera Actions")] -> w80
              tunnel: [w102 w104] -> w79
              tunnel: "Orca Flash ROI" -> [w102 w104]
              frame "Get ROI", Default {
              }
              frame "Set ROI" {
              }
            }
            n134 = Bundle By Name(cluster=w73, "Running?"=FALSE, "Camera Actions"=w80, "sCMOS ROI"=w79) -> (w78:T6)
            n135 = Send Notification(notification=w78, notifier=w74) -> (notifier out=w77:refnum<notifier>)  [unwired: 1 in, 1 out]
            n136 = Wait on Notification(notifier=w77, ignore previous (F)=TRUE) -> (notification=w76:T6)  [unwired: 2 in, 3 out]
            n137 = Unbundle By Name(w76) -> ("sCMOS ROI"=w66:T1)
            n138 = local write "Orca Flash ROI"(w66) -> ()
          }
          event "Set Parameter", "Get Parameter": Value Change {
            n139 = event-data() -> ("CtlRef"=w121:refnum<vi>)  [unwired: 1 in, 1 out]
            n140 = Get Notifier Status(notifier=w110) -> (notifier out=w108:refnum<notifier>, current notification=w107:T6, # waiting=w106:i32)  [unwired: 1 in, 2 out]
            n141 = Equal To 0?(x=w106) -> (x = 0?=w109:bool)
            n142 = case shown="True" w109 {
              tunnel: w108 -> [w125 w134]
              tunnel: w107 -> [w124 w133]
              tunnel: [w125 w129] -> w113
              tunnel: [w124 w128] -> w112
              frame False {
              }
              frame True {
                n143 = Bundle By Name(cluster=w133, "Running?"=FALSE, "Camera Actions"=Orca_Flash_Actions."IDLE") -> (w131:T6)
                n144 = Send Notification(notification=w131, notifier=w134) -> (notifier out=w130:refnum<notifier>)  [unwired: 1 in, 1 out]
                n145 = for {
                  N: 2000 -> [_]
                  tunnel: w130 -> [w140]
                  tunnel: [w137] -> w129
                  tunnel: [w136] -> w128
                  stop <- w138 stop-if-true
                  n146 = Get Notifier Status(notifier=w140) -> (notifier out=w137:refnum<notifier>, current notification=w136:T6, # waiting=w139:i32)  [unwired: 1 in, 2 out]
                  n147 = Not Equal To 0?(x=w139) -> (x != 0?=w138:bool)
                  n148 = Wait (ms)(milliseconds to wait=u32 1) -> ()  [unwired: 1 out]
                }
              }
            }
            n149 = property class="Bool"(reference=w121) -> ("Label.Text"=w120:string)  [unwired: 1 in, 2 out]
            n150 = case shown="\"Set Parameter\"" w120 {
              tunnel: [Orca_Flash_Actions."GETPARAM" ("Camera Actions") Orca_Flash_Actions."SETPARAM" ("Camera Actions")] -> w119
              frame "Get Parameter", Default {
              }
              frame "Set Parameter" {
              }
            }
            n151 = Bundle By Name(cluster=w112, "sCMOS Parameter"="sCMOS Parameter", "Running?"=FALSE, "Camera Actions"=w119) -> (w118:T6)
            n152 = Send Notification(notification=w118, notifier=w113) -> (notifier out=w117:refnum<notifier>)  [unwired: 1 in, 1 out]
            n153 = Wait on Notification(notifier=w117, ignore previous (F)=TRUE) -> (notification=w116:T6)  [unwired: 2 in, 3 out]
            n154 = Unbundle By Name(w116) -> ("sCMOS Parameter"=w115:T2)
            n155 = local write "sCMOS Parameter"(w115) -> ()
          }
          event "PREVIEW", "RECORD": Value Change {
            n156 = event-data() -> ("CtlRef"=w157:refnum<vi>, "NewVal"=w155:bool)  [unwired: 1 in, 1 out]
            n157 = Get Notifier Status(notifier=w153) -> (notifier out=w145:refnum<notifier>, current notification=w144:T6, # waiting=w143:i32)  [unwired: 1 in, 2 out]
            n158 = Equal To 0?(x=w143) -> (x = 0?=w146:bool)
            n159 = property class="Bool (strict)"(reference=w157) -> ("Label.Text"=w156:string)  [unwired: 1 in, 2 out]
            n160 = case shown="True" w146 {
              tunnel: w145 -> [w160 w169]
              tunnel: [w160 w165] -> w148
              tunnel: [w159 w163] -> w147
              tunnel: w144 -> [w159 w162]
              frame False {
              }
              frame True {
                n161 = Bundle By Name(cluster=w162, "Running?"=FALSE, "Camera Actions"=Orca_Flash_Actions."IDLE") -> (w167:T6)
                n162 = Send Notification(notification=w167, notifier=w169) -> (notifier out=w166:refnum<notifier>)  [unwired: 1 in, 1 out]
                n163 = for {
                  N: 2000 -> [_]
                  tunnel: w166 -> [w175]
                  tunnel: [w174] -> w165
                  tunnel: [w173] -> w163
                  stop <- w171 stop-if-true
                  n164 = Get Notifier Status(notifier=w175) -> (notifier out=w174:refnum<notifier>, current notification=w173:T6, # waiting=w172:i32)  [unwired: 1 in, 2 out]
                  n165 = Not Equal To 0?(x=w172) -> (x != 0?=w171:bool)
                  n166 = Wait (ms)(milliseconds to wait=u32 1) -> ()  [unwired: 1 out]
                }
              }
            }
            n167 = case shown="\"PREVIEW\"" w156 {
              tunnel: w155 -> [w178 _ w188]
              tunnel: [w177 FALSE w187] -> w151
              tunnel: [w176 Orca_Flash_Actions."IDLE" ("Camera Actions") w186] -> w154
              frame "PREVIEW" {
                n168 = case shown="False" w178 {
                  selector: w178 -> [_ w183]
                  tunnel: [FALSE w182] -> w177
                  tunnel: [Orca_Flash_Actions."IDLE" ("Camera Actions") Orca_Flash_Actions."PREVIEW" ("Camera Actions")] -> w176
                  frame False {
                  }
                  frame True {
                    n169 = Not(x=w183) -> (.not. x?=w182:bool)
                    n170 = local write "RECORD"(w182) -> ()
                  }
                }
              }
              frame Default {
              }
              frame "RECORD" {
                n171 = case shown="True" w188 {
                  selector: w188 -> [_ w193]
                  tunnel: [FALSE w192] -> w187
                  tunnel: [Orca_Flash_Actions."IDLE" ("Camera Actions") Orca_Flash_Actions."RECORD" ("Camera Actions")] -> w186
                  frame False {
                  }
                  frame True {
                    n172 = Not(x=w193) -> (.not. x?=w192:bool)
                    n173 = local write "PREVIEW"(w192) -> ()
                  }
                }
              }
            }
            n174 = Bundle By Name(cluster=w147, "# of frames"="# of frames", "Save Path"="Path", "Running?"=w151, "Camera Actions"=w154) -> (w152:T6)
            n175 = Send Notification(notification=w152, notifier=w148) -> ()  [unwired: 1 in, 2 out]
          }
          event "Sensor Mode", "Internal Line Interval Setpoint", "Number of lines": Value Change {
            n176 = event-data() -> ()  [unwired: 1 in, 6 out]
            n177 = Get Notifier Status(notifier=w201) -> (notifier out=w204:refnum<notifier>, current notification=w203:T6, # waiting=w202:i32)  [unwired: 1 in, 2 out]
            n178 = Equal To 0?(x=w202) -> (x = 0?=w205:bool)
            n179 = case shown="True" w205 {
              tunnel: w204 -> [w209 w218]
              tunnel: w203 -> [w208 w217]
              tunnel: [w209 w213] -> w200
              tunnel: [w208 w212] -> w199
              frame False {
              }
              frame True {
                n180 = Bundle By Name(cluster=w217, "Running?"=FALSE, "Camera Actions"=Orca_Flash_Actions."IDLE") -> (w215:T6)
                n181 = Send Notification(notification=w215, notifier=w218) -> (notifier out=w214:refnum<notifier>)  [unwired: 1 in, 1 out]
                n182 = for {
                  N: 2000 -> [_]
                  tunnel: w214 -> [w224]
                  tunnel: [w221] -> w213
                  tunnel: [w220] -> w212
                  stop <- w222 stop-if-true
                  n183 = Get Notifier Status(notifier=w224) -> (notifier out=w221:refnum<notifier>, current notification=w220:T6, # waiting=w223:i32)  [unwired: 1 in, 2 out]
                  n184 = Not Equal To 0?(x=w223) -> (x != 0?=w222:bool)
                  n185 = Wait (ms)(milliseconds to wait=u32 1) -> ()  [unwired: 1 out]
                }
              }
            }
            n186 = case shown="\"Progressive\"" "Sensor Mode" {
              tunnel: [Orca_Flash_Actions."AREA MODE" ("Camera Actions") Orca_Flash_Actions."PROGRESSIVE MODE" ("Camera Actions")] -> w195
              frame "Area", Default {
              }
              frame "Progressive" {
              }
            }
            n187 = Bundle By Name(cluster=w199, "Running?"=FALSE, "Camera Actions"=w195) -> (w194:T6)
            n188 = Send Notification(notification=w194, notifier=w200) -> ()  [unwired: 1 in, 2 out]
          }
          event "Use Display Module": Value Change {
            n189 = event-data() -> ("NewVal"=w226:bool)  [unwired: 1 in]
            n190 = Get Notifier Status(notifier=w225) -> (current notification=w227:T6)  [unwired: 1 in, 4 out]
            n191 = Unbundle By Name(w227) -> ("Image Ref"=w241:T8)
            n192 = Obtain Notifier(name (unnamed)="Display Module IMAQ Refs", notification data type=T8[] [], create if not found? (T)=FALSE) -> (notifier out=w234:refnum<notifier>, error out=w235:errorcluster)  [unwired: 1 in, 1 out]
            n193 = Get Notifier Status(notifier=w234, error in (no error)=w235) -> (notifier out=w233:refnum<notifier>, current notification=w231:T8[], error out=w232:errorcluster)  [unwired: 2 out]
            n194 = case shown="False" w226 {
              tunnel: w233 -> [w250 w260]
              tunnel: w232 -> [w244 w259]
              tunnel: w231 -> [w246 w262]
              tunnel: [w245 w261] -> w228
              tunnel: [w250 w260] -> w230
              tunnel: [w244 w259] -> w229
              tunnel: w241 -> [w243 w258]
              frame False {
                n195 = Equal?(x=w246, y=w243) -> (x = y?=w249:bool[])
                n196 = for {
                  tunnel: w249 -> [w257] mode=indexing
                  tunnel: [w256] -> w247
                  i -> [w256]
                  stop <- w257 stop-if-true
                }
                n197 = Or Array Elements(Boolean array=w249) -> (logical OR=w248:bool)
                n198 = case shown="True" w248 {
                  tunnel: w247 -> [_ w254]
                  tunnel: w246 -> [w251 w253]
                  tunnel: [w251 w252] -> w245
                  frame False {
                  }
                  frame True {
                    n199 = Delete From Array(array=w253, length=1, index=w254) -> (array with subset deleted=w252:T8[])  [unwired: 1 out]
                  }
                }
              }
              frame True {
                n200 = Build Array (concatenate)(w262, w258) -> (w261:T8[])
              }
            }
            n201 = Send Notification(notification=w228, notifier=w230, error in (no error)=w229) -> (notifier out=w236:refnum<notifier>, error out=w237:errorcluster)
            n202 = Release Notifier(notifier=w236, error in (no error)=w237) -> ()  [unwired: 1 in, 3 out]
          }
          event "QUIT": Value Change {
            n203 = event-data() -> ("NewVal"=w273:bool)  [unwired: 1 in]
            n204 = Get Notifier Status(notifier=w269) -> (notifier out=w265:refnum<notifier>, current notification=w264:T6, # waiting=w263:i32)  [unwired: 1 in, 2 out]
            n205 = Equal To 0?(x=w263) -> (x = 0?=w266:bool)
            n206 = case shown="True" w266 {
              tunnel: w265 -> [w275 w280]
              tunnel: [w275 w278] -> w268
              tunnel: [w274 w277] -> w267
              tunnel: w264 -> [w274 w276]
              frame False {
              }
              frame True {
                n207 = Bundle By Name(cluster=w276, "Running?"=FALSE, "Camera Actions"=Orca_Flash_Actions."IDLE") -> (w279:T6)
                n208 = Send Notification(notification=w279, notifier=w280) -> (notifier out=w283:refnum<notifier>)  [unwired: 1 in, 1 out]
                n209 = for {
                  N: 2000 -> [_]
                  tunnel: w283 -> [w290]
                  tunnel: [w287] -> w278
                  tunnel: [w286] -> w277
                  stop <- w288 stop-if-true
                  n210 = Get Notifier Status(notifier=w290) -> (notifier out=w287:refnum<notifier>, current notification=w286:T6, # waiting=w289:i32)  [unwired: 1 in, 2 out]
                  n211 = Not Equal To 0?(x=w289) -> (x != 0?=w288:bool)
                  n212 = Wait (ms)(milliseconds to wait=u32 1) -> ()  [unwired: 1 out]
                }
              }
            }
            n213 = Bundle By Name(cluster=w267, "Running?"=FALSE, "Camera Actions"=Orca_Flash_Actions."QUIT") -> (w272:T6)
            n214 = Send Notification(notification=w272, notifier=w268) -> ()  [unwired: 1 in, 2 out]
          }
        }
      }
      n215 = Release Notifier(notifier=w31, force destroy? (F)=TRUE) -> ()  [unwired: 1 in, 3 out]
    }
    frame Error {
      n216 = call <userlib>:"tm_deinitialize_40.vi"("error in (no error)"=w591) -> ("error out"=w583:errorcluster)  [unwired: 10 in]
      n217 = Release Notifier(notifier=w584, force destroy? (F)=TRUE, error in (no error)=w583) -> (error out=w582:errorcluster)  [unwired: 2 out]
      n218 = Unbundle By Name(w582) -> ("source"=w586:string)
      n219 = call <vilib>:"Space Constant.vi"() -> ("String"=w589:string)
      n220 = Concatenate Strings(w581, w589, "Device Error." ("string"), "\r", w586) -> (w590:string)
      n221 = One Button Dialog(message=w590) -> ()  [unwired: 1 in, 1 out]
    }
  }
